vi "type pun.vi"() -> ()   [LabVIEW 2017]
panel:
  out "*(type *) &x":sgl
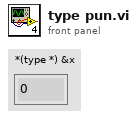
[diagram p1: front panel]
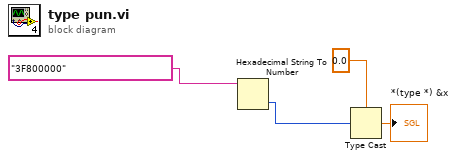
[diagram p0: block diagram]
diagram:
  n1 = Hexadecimal String To Number(string="3F800000") -> (number=w3:u32)  [unwired: 2 in, 1 out]
  n2 = Type Cast(type=sgl 0.0, x=w3) -> (*(type *) &x=→"*(type *) &x":sgl)
